vi "Read Holding Registers.vi"(8 "error in":errorcluster, 9 "number of inputs":u16, 10 "starting address":u16, 11 "Modbus slave in":refnum<class "Modbus Slave.lvclass">) -> (0 "error out":errorcluster, 2 "register values":u16[](array[numeric]), 3 "Modbus slave out":refnum<class "Modbus Slave.lvclass">)   [LabVIEW 2012, in "Modbus Slave.lvclass"]
doc: "Reads <B>number of inputs</B> holding registers starting at <B>starting address</B> from the device."
uses:
  Modbus Slave.lvclass
  Modbus Slave.lvclass/Modbus Slave.ctl
  Data Model/Device Data Model.lvclass
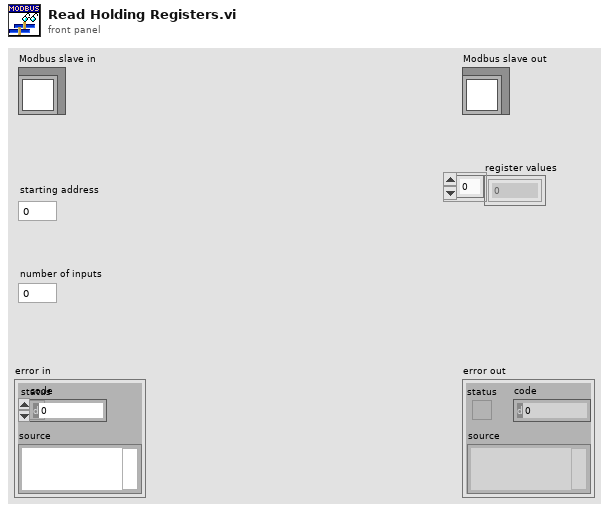
[diagram p1: front panel]
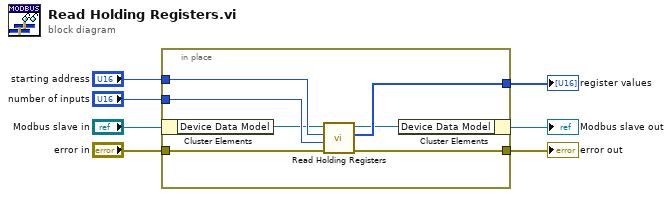
[diagram p0: block diagram]
diagram:
  n1 = in-place {
    in-place-border: [w14] -> w5
    in-place-border: "number of inputs" -> [w13]
    in-place-border: "starting address" -> [w12]
    in-place-border: [w11] -> w7
    in-place-border: "error in" -> [w10]
    n2 = in-place-cluster #1("Modbus slave in") -> ("Device Data Model"=w8:refnum<class "Device Data Model.lvclass">)
    n3 = call-dynamic "Read Holding Registers.vi"("error in"=w10, "number of registers"=w13, "starting address"=w12, "device data model in"=w8) -> ("error out"=w11:errorcluster, "data"=w14:u16[], "device data model out"=w9:refnum<class "Device Data Model.lvclass">)  [unwired: 5 in]
    n4 = in-place-cluster #1("Device Data Model"=w9) -> (→"Modbus slave out":refnum<class "Modbus Slave.lvclass">)
  }
  "error out" <- w7
  "register values" <- w5
